vi "AcqFond_FGV.vi"(8 "Error In":errorcluster, 9 "Image":u16[][](array[numeric]), 10 "Cluster":cluster{"nbLine":i32, "nbCol":i32, "nbrIma":i32}, 11 "Enum":enum16{"Init", "Add", "Close"}(ring)) -> (0 "Error Out":errorcluster, 3 "fond":dbl[][](array[numeric]))   [LabVIEW 2020]
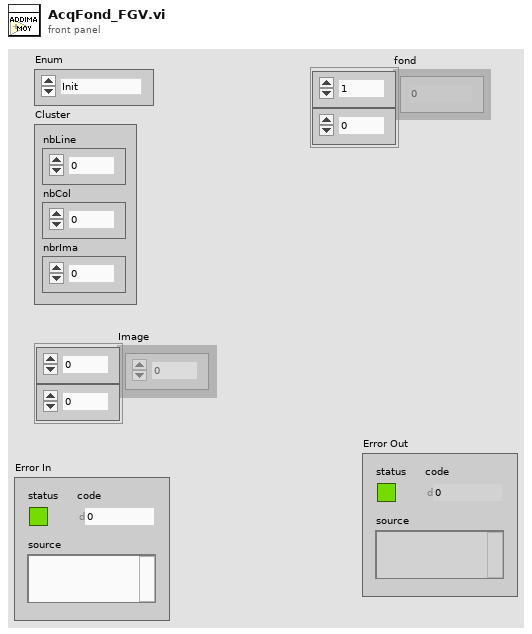
[diagram p1: front panel]
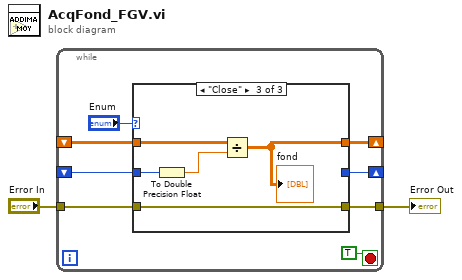
[diagram p0: block diagram]
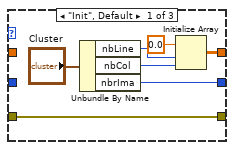
[diagram p2: hidden frame]
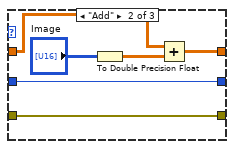
[diagram p3: hidden frame]
diagram:
  n1 = while {
    shift-right: [w9] -> _
    shift-left: _ -> [w8]
    tunnel: "Error In" -> [w6]
    tunnel: [w5] -> w1
    shift-right: [w4] -> _
    shift-left: _ -> [w3]
    stop <- TRUE stop-if-true
    n2 = case shown="\"Close\"" "Enum" {
      tunnel: [w17 w22 w26] -> w9
      tunnel: w8 -> [_ w23 w28]
      tunnel: w6 -> [w12 w19 w25]
      tunnel: [w12 w19 w25] -> w5
      tunnel: [w11 w18 _] -> w4
      tunnel: w3 -> [_ w18 w24]
      frame "Init", Default {
        n3 = Unbundle By Name("Cluster") -> ("nbLine"=w14:i32, "nbCol"=w13:i32, "nbrIma"=w11:i32)
        n4 = Initialize Array(0.0 ("element"), w14, w13) -> (w17:dbl[][])
      }
      frame "Add" {
        n5 = To Double Precision Float(number="Image") -> (double precision float=w20:dbl[][])
        n6 = Add(x=w23, y=w20) -> (x+y=w22:dbl[][])
      }
      frame "Close" {
        n7 = To Double Precision Float(number=w24) -> (double precision float=w27:dbl)
        n8 = Divide(x=w28, y=w27) -> (x/y=w26:dbl[][])
        "fond" <- w26
      }
    }
  }
  "Error Out" <- w1
